vi "UI Array act All Buttons.vi"(8 "error in (no error)":errorcluster, 9 "Default Shunt Resistor":T1=enum."50 Ohms", 10 "KH All Buttons":T10(radio), 11 "UI Channels []":T2[](array[typedef]) {"KH"."Channel" items=["A 1"]}) -> (0 "error out":errorcluster, 3 "UI Channels [] out":T2[](array[typedef]) {"KH"."Channel" items=["A 1"]})   [LabVIEW 2016, in "Control Experiment UI.lvclass"]
uses:
  Control Experiment UI.lvclass
  <userlib>/LevyLab/Krohn Hite 7008/typedefs/Input Configuration-Enum.ctl
  <userlib>/LevyLab/Krohn Hite 7008/Instrument.KH7008.lvclass
  <userlib>/LevyLab/Krohn Hite 7008/typedefs/Shunt-Enum.ctl
  Typedefs/UI Channels.AI--Cluster.ctl
  Control Experiment/Private/Control Experiment SM/Typedefs/KH Mode-enum.ctl
  Control Experiment/Control Experiment.lvclass
  Typedefs/UI Channels.Device--Cluster.ctl
  <userlib>/LevyLab/Krohn Hite 7008/typedefs/Gain-Enum.ctl
  Typedefs/UI Channels.KH--Cluster.ctl
  Typedefs/UI Channels.AO--Cluster.ctl
  Typedefs/UI Channels--Cluster.ctl
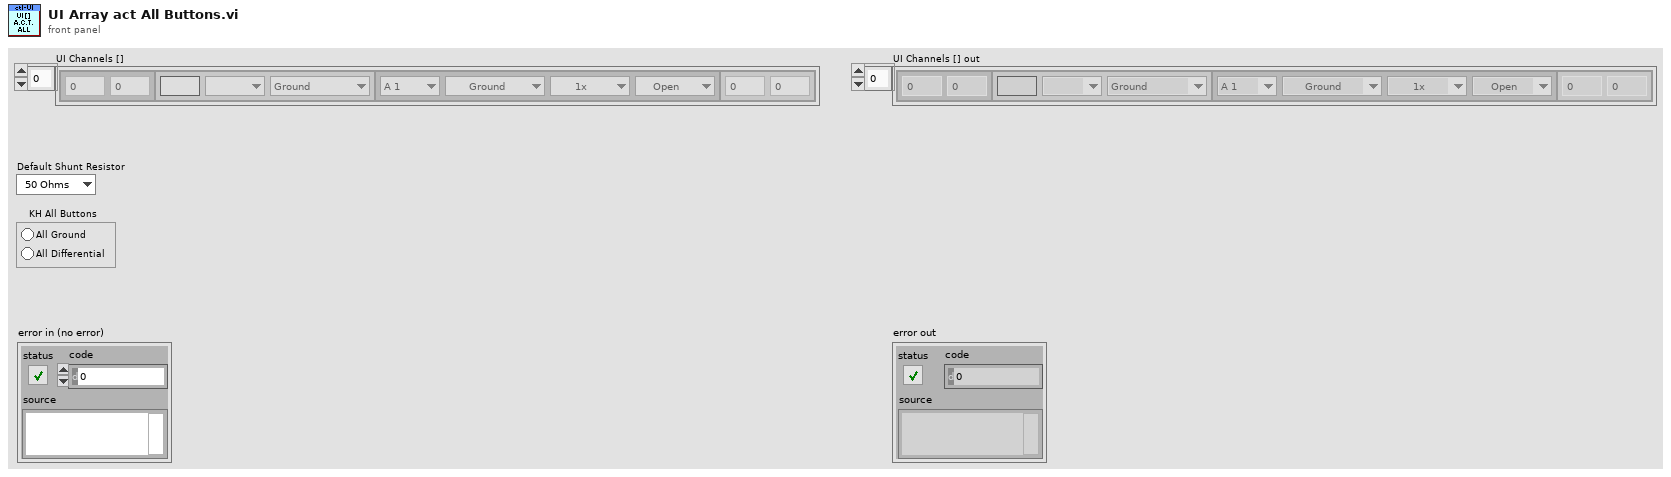
[diagram p1: front panel]
types:
  T1 = typedef "Instrument.KH7008.lvclass/Shunt-Enum.ctl" = enum16{"Open", "50 Ohms", "500 Ohms", "5k Ohms", "50k Ohms", "10M Ohm"}
  T2 = typedef "Control Experiment UI.lvclass/UI Channels--Cluster.ctl" = cluster{"AI":T3, "Device":T4, "KH":T6, "AO":T9}
  T3 = typedef "Control Experiment UI.lvclass/UI Channels.AI--Cluster.ctl" = cluster{"Channel":u32, "Gain":dbl}
  T4 = typedef "Control Experiment UI.lvclass/UI Channels.Device--Cluster.ctl" = cluster{"Electrode":string, "Configuration":T5, "Label":u16}
  T5 = typedef "Control Experiment.lvclass/KH Mode-enum.ctl" = enum16{"Ground", "Current", "Voltage (SE)", "Voltage (Diff)", "Gate"}
  T6 = typedef "Control Experiment UI.lvclass/UI Channels.KH--Cluster.ctl" = cluster{"Channel":u16, "Configuration":T7, "Gain":T8, "Shunt Resistor":T1}
  T7 = typedef "Instrument.KH7008.lvclass/Input Configuration-Enum.ctl" = enum16{"Ground", "SE+ (-gnd)", "SE- (+gnd)", "Differential"}
  T8 = typedef "Instrument.KH7008.lvclass/Gain-Enum.ctl" = enum16{"1x", "10x", "100x", "1000x"}
  T9 = typedef "Control Experiment UI.lvclass/UI Channels.AO--Cluster.ctl" = cluster{"Channel":u32, "Gain":dbl}
  T10 = enum32{"No Selection", "All Ground", "All Differential"}
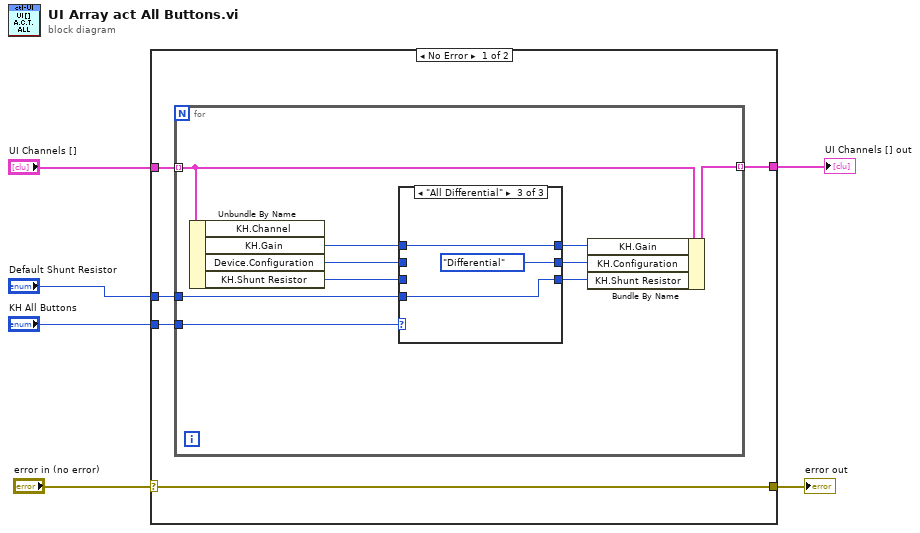
[diagram p0: block diagram]
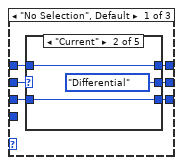
[diagram p2: hidden frame]
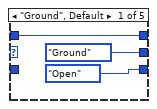
[diagram p3: hidden frame]
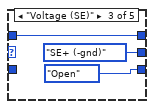
[diagram p4: hidden frame]
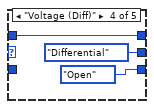
[diagram p5: hidden frame]
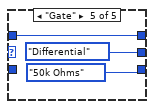
[diagram p6: hidden frame]
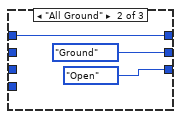
[diagram p7: hidden frame]
diagram:
  n1 = case shown="No Error" "error in (no error)" {
    selector: "error in (no error)" -> [w7 w50]
    tunnel: "KH All Buttons" -> [w11 _]
    tunnel: [w10 w49] -> w5
    tunnel: "UI Channels []" -> [w9 w49]
    tunnel: "Default Shunt Resistor" -> [w8 _]
    tunnel: [w7 w50] -> w1
    frame No Error {
      n2 = for {
        tunnel: w9 -> [w20] mode=indexing
        tunnel: [w21] -> w10 mode=indexing
        tunnel: w11 -> [w17]
        tunnel: w8 -> [w12]
        n3 = Unbundle By Name(w20) -> ("KH.Gain"=w19:T8, "Device.Configuration"=w16:T5, "KH.Shunt Resistor"=w15:T1)  [unwired: 1 out]
        n4 = case shown="\"All Differential\"" w17 {
          tunnel: w16 -> [w23 _ _]
          tunnel: [w27 Input_Configuration-Enum."Ground" ("Input Config") Input_Configuration-Enum."Differential" ("Input Config")] -> w14
          tunnel: w19 -> [w26 w45 w48]
          tunnel: [w25 w45 w48] -> w18
          tunnel: [w24 Shunt-Enum."Open" ("Shunt Resistor") w46] -> w13
          tunnel: w15 -> [w22 _ _]
          tunnel: w12 -> [_ _ w46]
          frame "No Selection", Default {
            n5 = case shown="\"Current\"" w23 {
              tunnel: [Input_Configuration-Enum."Ground" ("Input Config") Input_Configuration-Enum."Differential" ("Input Config") Input_Configuration-Enum."SE+ (-gnd)" ("Input Config") Input_Configuration-Enum."Differential" ("Input Config") Input_Configuration-Enum."Differential" ("Input Config")] -> w27
              tunnel: [Shunt-Enum."Open" ("Shunt Resistor") w31 Shunt-Enum."Open" ("Shunt Resistor") Shunt-Enum."Open" ("Shunt Resistor") Shunt-Enum."50k Ohms" ("Shunt Resistor")] -> w24
              tunnel: w26 -> [w28 w32 w35 w39 w41]
              tunnel: [w28 w32 w35 w39 w41] -> w25
              tunnel: w22 -> [_ w31 _ _ _]
              frame "Ground", Default {
              }
              frame "Current" {
              }
              frame "Voltage (SE)" {
              }
              frame "Voltage (Diff)" {
              }
              frame "Gate" {
              }
            }
          }
          frame "All Ground" {
          }
          frame "All Differential" {
          }
        }
        n6 = Bundle By Name(cluster=w20, "KH.Gain"=w18, "KH.Configuration"=w14, "KH.Shunt Resistor"=w13) -> (w21:T2)
      }
    }
    frame Error {
    }
  }
  "UI Channels [] out" <- w5
  "error out" <- w1
